vi "ConfDB-GFV.vi"(8 "error in (no error)":errorcluster, 10 "Data in":variant, 11 "Command In":T1=enum."Configure DB") -> (0 "error out":errorcluster, 2 "Data out":variant)   [LabVIEW 2013]
uses:
  ConfEnum.ctl
  ConfDB.ctl
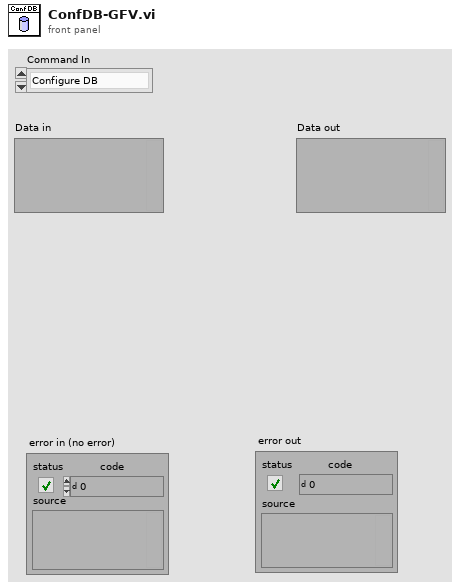
[diagram p1: front panel]
types:
  T1 = typedef "ConfEnum.ctl" = enum16{"Init", "GetFileNameStartIndex", "Configure DB"}
  T2 = typedef "ConfDB.ctl" = cluster{"NumberOfImages":i32, "NoImages2SaveAroundFreeze":i32, "Path":path, "NameOfPartialFile":string, "StartIndex":i32, "NumberOfStdTol":i32}
  T3 = cluster{"NumberOfImages":i32, "Path":path, "NameOfPartialFile":string, "StartIndex":i32}
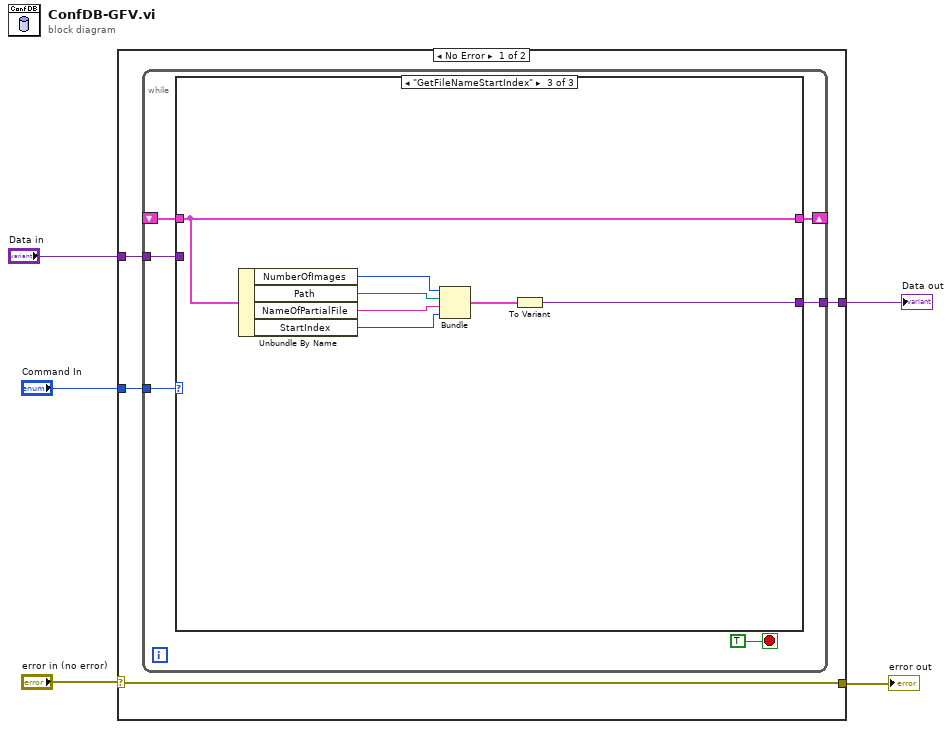
[diagram p0: block diagram]
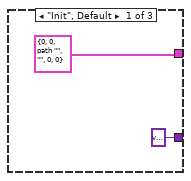
[diagram p2: hidden frame]
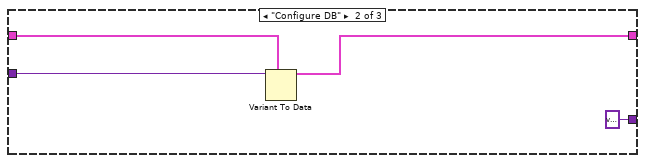
[diagram p3: hidden frame]
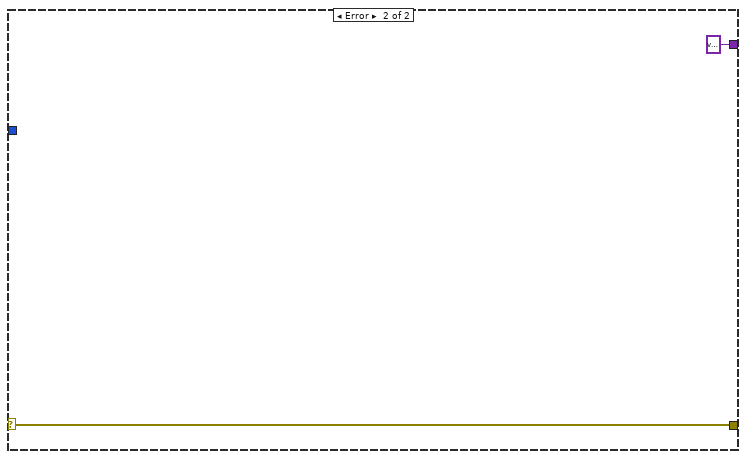
[diagram p4: hidden frame]
diagram:
  n1 = case shown="No Error" "error in (no error)" {
    selector: "error in (no error)" -> [w9 w30]
    tunnel: [w9 w30] -> w4
    tunnel: "Command In" -> [w8 _]
    tunnel: "Data in" -> [w7 _]
    tunnel: [w6 variant ("Variant")] -> w1
    frame No Error {
      n2 = while {
        tunnel: w8 -> [w14]
        shift-right: [w13] -> _
        shift-left: _ -> [w11]
        tunnel: w7 -> [w12]
        tunnel: [w10] -> w6
        stop <- TRUE stop-if-true
        n3 = case shown="\"GetFileNameStartIndex\"" w14 {
          tunnel: [T2 {"NumberOfImages"=0, "NoImages2SaveAroundFreeze"=0, "Path"=path "", "NameOfPartialFile"="", "StartIndex"=0, "NumberOfStdTol"=0} ("ConfDB") w19 w27] -> w13
          tunnel: w12 -> [_ w21 _]
          tunnel: w11 -> [_ w20 w27]
          tunnel: [variant ("Variant") variant ("Variant") w28] -> w10
          frame "Init", Default {
          }
          frame "Configure DB" {
            n4 = Variant To Data(type=w20, Variant=w21) -> (data=w19:T2)  [unwired: 1 in, 1 out]
          }
          frame "GetFileNameStartIndex" {
            n5 = Unbundle By Name(w27) -> ("NumberOfImages"=w26:i32, "Path"=w25:path, "NameOfPartialFile"=w24:string, "StartIndex"=w23:i32)
            n6 = Bundle("NumberOfImages"=w26, "Path"=w25, "NameOfPartialFile"=w24, "StartIndex"=w23) -> (w22:T3)  [unwired: 1 in]
            n7 = To Variant(anything=w22) -> (Variant=w28:variant)
          }
        }
      }
    }
    frame Error {
    }
  }
  "error out" <- w4
  "Data out" <- w1
